vi "DistanciaRoboInimigoBola.vi"(8 "Y bola":dbl format="%#_13g", 9 "X bola":dbl format="%#_13g", 10 "Y inimigo":dbl format="%#_13g", 11 "X inimigo":dbl format="%#_13g") -> (0 "Y inimigo":dbl format="%#_13g", 1 "X inimigo":dbl format="%#_13g", 3 "Distância":dbl format="%#_13g")   [LabVIEW 2017]
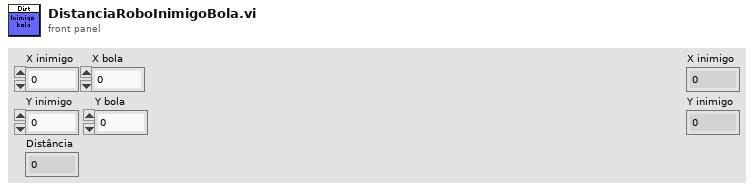
[diagram p1: front panel]
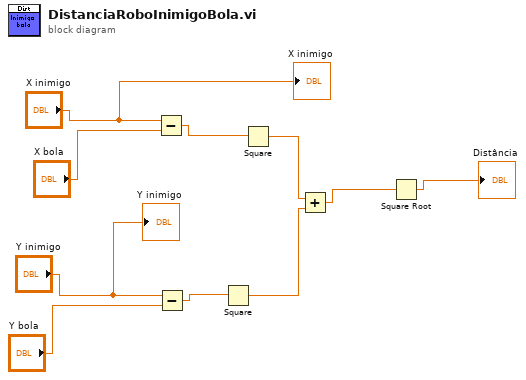
[diagram p0: block diagram]
diagram:
  n1 = Subtract(x="X inimigo", y="X bola") -> (x-y=w8:dbl)
  n2 = Subtract(x="Y inimigo", y="Y bola") -> (x-y=w7:dbl)
  n3 = Square(x=w7) -> (x^2=w5:dbl)
  n4 = Square(x=w8) -> (x^2=w6:dbl)
  n5 = Add(x=w6, y=w5) -> (x+y=w4:dbl)
  n6 = Square Root(x=w4) -> (sqrt(x)=→"Distância":dbl)
  "X inimigo" <- "X inimigo"
  "Y inimigo" <- "Y inimigo"
